vi "Lookup State.vi"(8 "error in (no error)":errorcluster, 10 "State":string, 11 "Sequence Config in":refnum<class "Sequence Config.lvclass">) -> (0 "error out":errorcluster, 2 "Info":T1, 3 "Sequence Config out":refnum<class "Sequence Config.lvclass">)   [LabVIEW 2023, in "VolatusSeqConfig.lvlib" / "Sequence Config.lvclass"]
uses:
  Sequence Config.lvclass
  State.ctl
  Step.ctl
  Command Config/Command Config.lvclass
  Transition Config/Transition Config.lvclass
  Debug Flags.ctl
  Sequence Config.lvclass/Sequence Config.ctl
  VolatusSeqConfig.lvlib
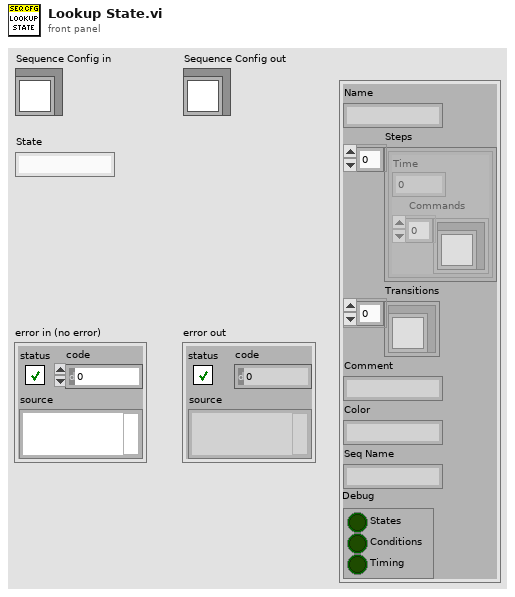
[diagram p1: front panel]
types:
  T1 = typedef "VolatusSeqConfig.lvlib/State.ctl" = cluster{"Name":string, "Steps":T2[], "Transitions":refnum<class "Transition Config.lvclass">[], "Comment":string, "Color":string, "Seq Name":string, "Debug":T3}
  T2 = typedef "VolatusSeqConfig.lvlib/Step.ctl" = cluster{"Time":dbl, "Commands":refnum<class "Command Config.lvclass">[]}
  T3 = typedef "VolatusSeqConfig.lvlib/Debug Flags.ctl" = cluster{"States":bool, "Conditions":bool, "Timing":bool}
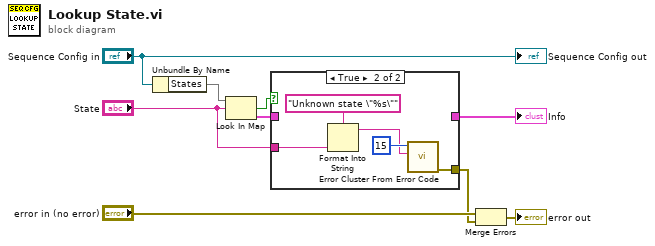
[diagram p0: block diagram]
diagram:
  n1 = Unbundle By Name("Sequence Config in") -> ("States"=w7:map{string, T1})
  n2 = Look In Map(map=w7, key="State") -> (key not found?=w6:bool, value=w5:T1)  [unwired: 1 in]
  n3 = case shown="True" w6 {
    tunnel: w5 -> [w10 _]
    tunnel: [w10 _] -> w4
    tunnel: "State" -> [_ w12]
    tunnel: [_ w11] -> w1
    frame False {
    }
    frame True {
      n4 = Format Into String(format string="Unknown state \"%s\"", w12) -> (resulting string=w13:string)  [unwired: 2 in, 1 out]
      n5 = call <vilib>:"Error Cluster From Error Code.vi"("error message (\"\")"=w13, "error code (0)"=15) -> ("error out"=w11:errorcluster)  [unwired: 7 in]
    }
  }
  "Info" <- w4
  n6 = Merge Errors("error in (no error)", w1) -> (→"error out":errorcluster)
  "Sequence Config out" <- "Sequence Config in"
